vi "PICOTEST M351XA Series Read Multiple.vi"() -> ()   [LabVIEW 2020]
doc: "This example shows how to configure the measurement function and take multiple readings."
uses:
  Public/Data/Read (Multiple Points).vi
  PICOTEST M351XA Series.lvlib
panel:
  out "Measurements":dbl[](array[numeric])
  in  "Timeout (10000 ms)":i32=10000 format="%#.6g"
  in  "Sample Count (25)":i32=25 min=1 max=50000
  in  "Function (0: DC Voltage)":u16(ring) items=["DC Voltage", "AC Voltage", "DC Current", "AC Current", "2W Resistance", "4W Resistance", "Frequency", "Period", "Continuity", "Diode", "VDC Ratio", "Temperature", "TCouple", "Capacitance"]
  in  "VISA resource name":refnum<visa-resource-name>
  # "(c) 2009 PICOTEST CORP.  ALL RIGHTS RESERVED."
  # "Read Multiple example shows how to select a function, \nuse a bus trigger, assign Sample Count, assigned the Timeout duration and fetch measurements.The Picotest M3511A does not support TCouple Function.\n\nInstructions:\n1. Select the working device on the VISA resource name.\n2. Select the working function and the other items for the\n    test control.\n3. Run the VI to take the measurements."
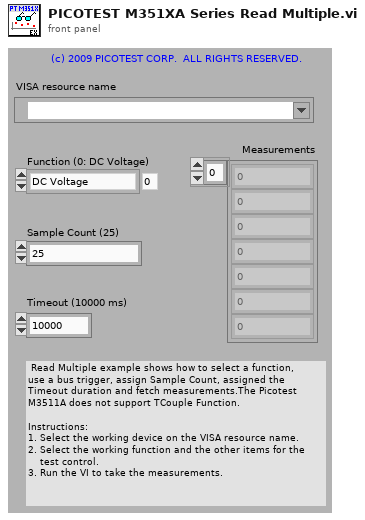
[diagram p1: front panel]
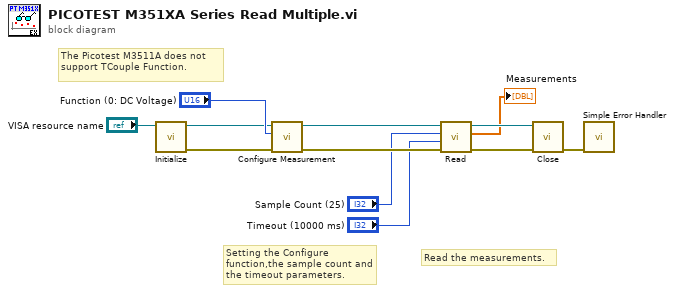
[diagram p0: block diagram]
diagram:
  # "The Picotest M3511A does not support TCouple Function."
  # "Read the measurements."
  # "Setting the Configure function,the sample count and the timeout parameters."
  n1 = call "Initialize.vi"("VISA resource name"="VISA resource name") -> ("error out"=w8:errorcluster, "VISA resource name out"=w9:refnum<visa-resource-name>)  [unwired: 9 in]
  n2 = call "Configure Measurement.vi"("error in (no error)"=w8, "Function ( 0:DC Voltage)"="Function (0: DC Voltage)", "VISA Resource Name"=w9) -> ("error out"=w6:errorcluster, "VISA resource name out"=w7:refnum<visa-resource-name>)  [unwired: 7 in]
  n3 = call-poly "Read.vi"("error in (no error)"=w6, "Timeout (10000 ms)"="Timeout (10000 ms)", "Sample Count (1)"="Sample Count (25)", "VISA resource name"=w7) -> ("error out"=w4:errorcluster, "Measurements"=→"Measurements":dbl[], "VISA resource name out"=w5:refnum<visa-resource-name>)  [unwired: 5 in]
  n4 = call "Close.vi"("error in (no error)"=w4, "VISA resource name"=w5) -> ("error out"=w12:errorcluster)  [unwired: 9 in]
  n5 = call <vilib>:"Simple Error Handler.vi"("error in (no error)"=w12) -> ()  [unwired: 4 in, 5 out]
